vi "position.set.vi"(10 "Coordinates":T1, 11 "Fruit in":refnum<class "Fruit.lvclass">) -> (3 "Fruit out":refnum<class "Fruit.lvclass">)   [LabVIEW 2020, in "Fruit.lvclass"]
uses:
  Fruit.lvclass
  Snake/Type Defs/Coordinates.ctl
  Fruit.lvclass/Fruit.ctl
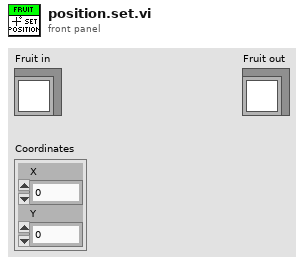
[diagram p1: front panel]
types:
  T1 = typedef "Coordinates.ctl" = cluster{"X":i32, "Y":i32}
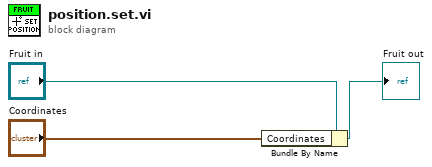
[diagram p0: block diagram]
diagram:
  n1 = Bundle By Name(cluster="Fruit in", "Coordinates"="Coordinates") -> (→"Fruit out":refnum<class "Fruit.lvclass">)
